vi "Animate two structures.vi"(4 "Atom Size":dbl=0.75, 6 "Scale":dbl(slide)=0.07482993197278912 scale=0.0..0.5, 8 "# Frames":i32(slide)=5 scale=0.0..100.0, 9 "Second Structure":T1, 10 "First Structure":T1, 11 "3D Plot Reference":refnum<vi>) -> ()   [LabVIEW 2010]
uses:
  <vilib>/Analysis/_algsub.llb/Real Vector Norm.vi
  <vilib>/Analysis/NI_AALPro.lvlib
  <vilib>/picture/3D Picture Control/NI_3D Picture Control.lvlib
panel:
  in  "Atomic Structure":refnum<vi>(3d-picture)
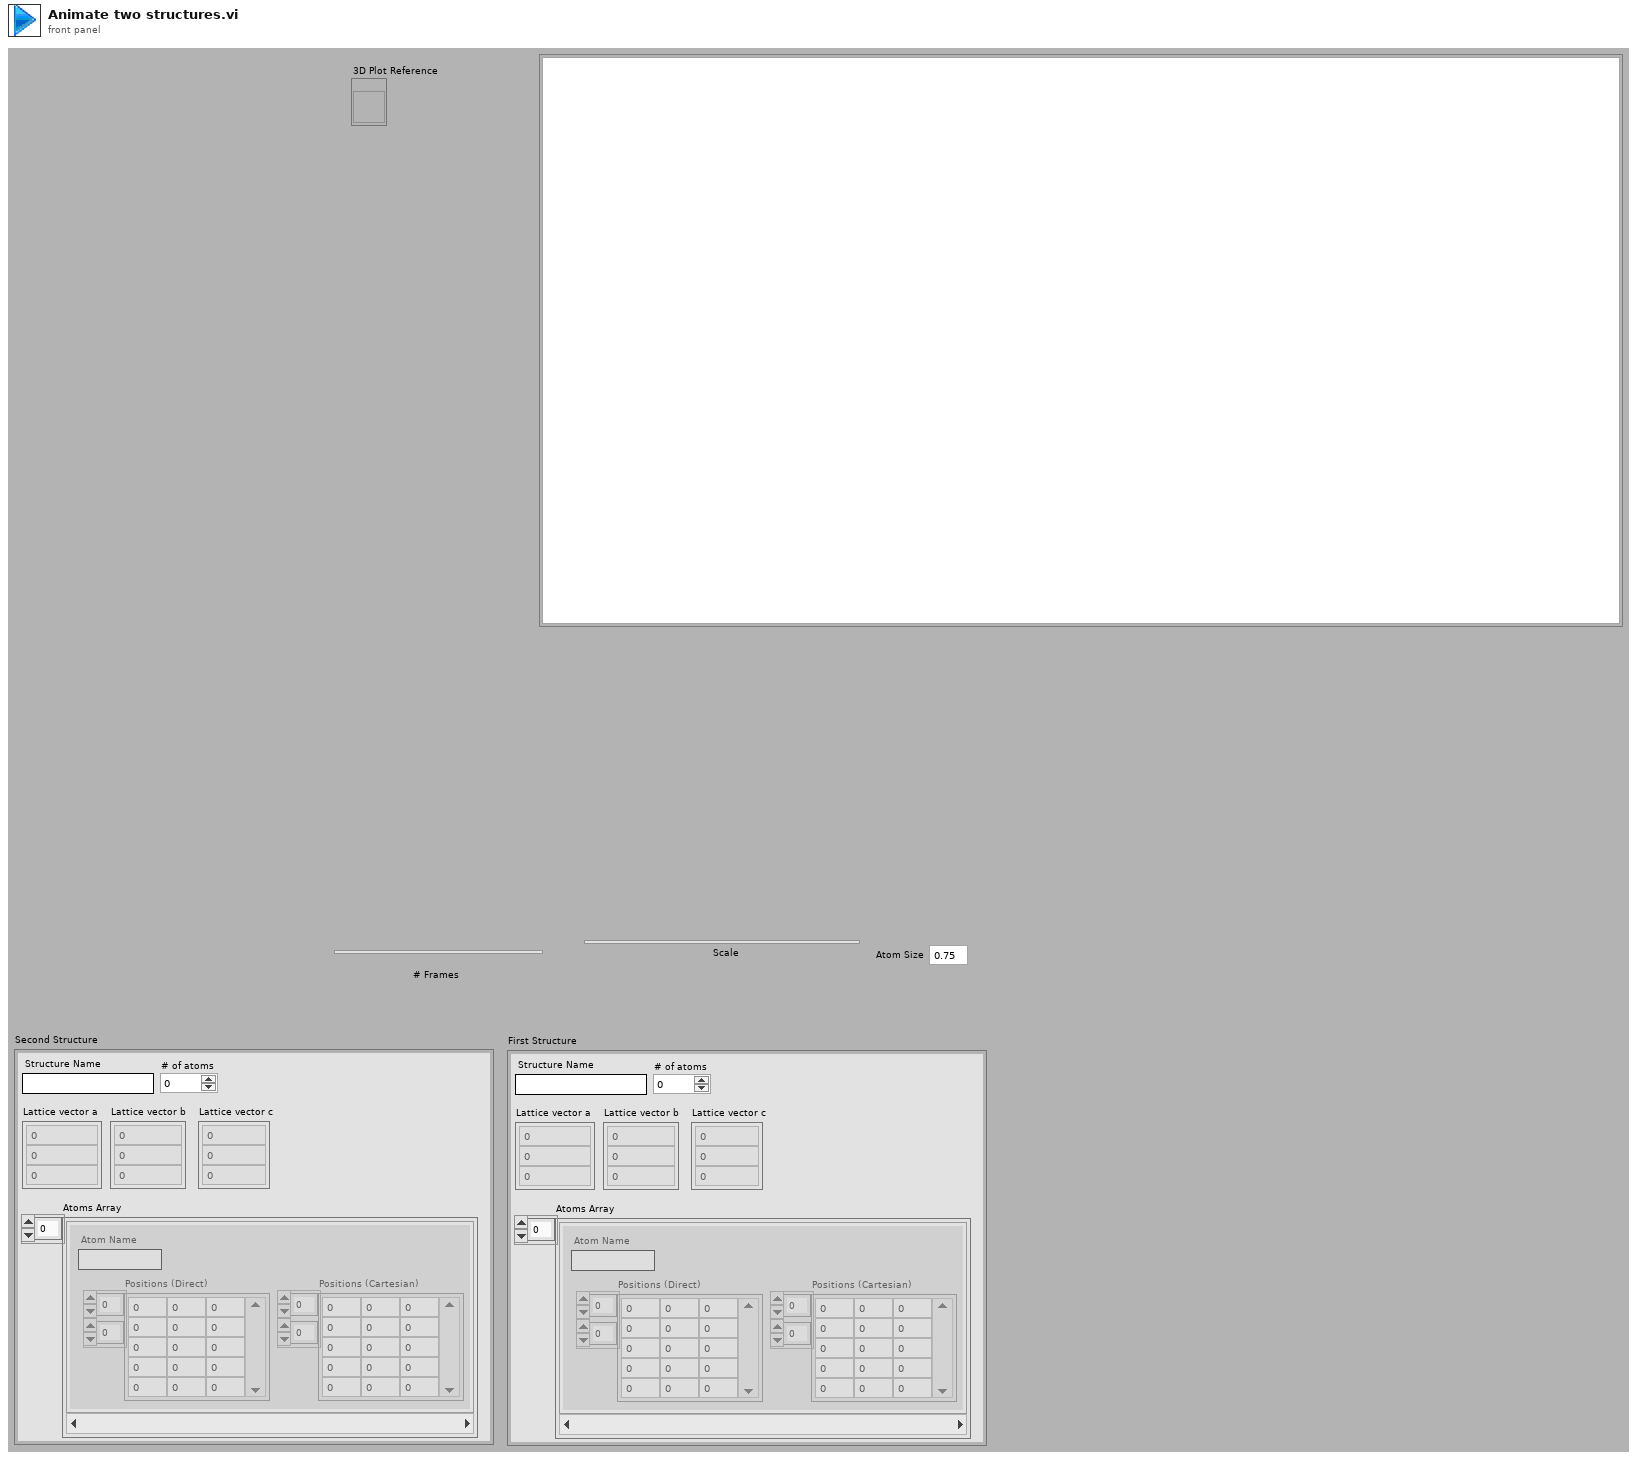
[diagram p1: front panel]
types:
  T1 = cluster{"Structure Name":string, "Lattice vector a":dbl[], "Lattice vector b":dbl[], "Lattice vector c":dbl[], "Atoms Array":cluster{"Atom Name":string, "Positions (Direct)":dbl[][], "Positions (Cartesian)":dbl[][]}[], "# of atoms":i32}
  T2 = cluster{"Red":sgl, "Green":sgl, "Blue":sgl, "Alpha":sgl}[]
  T3 = cluster{"Atom Name":string, "Positions (Direct)":dbl[][], "Positions (Cartesian)":dbl[][]}[]
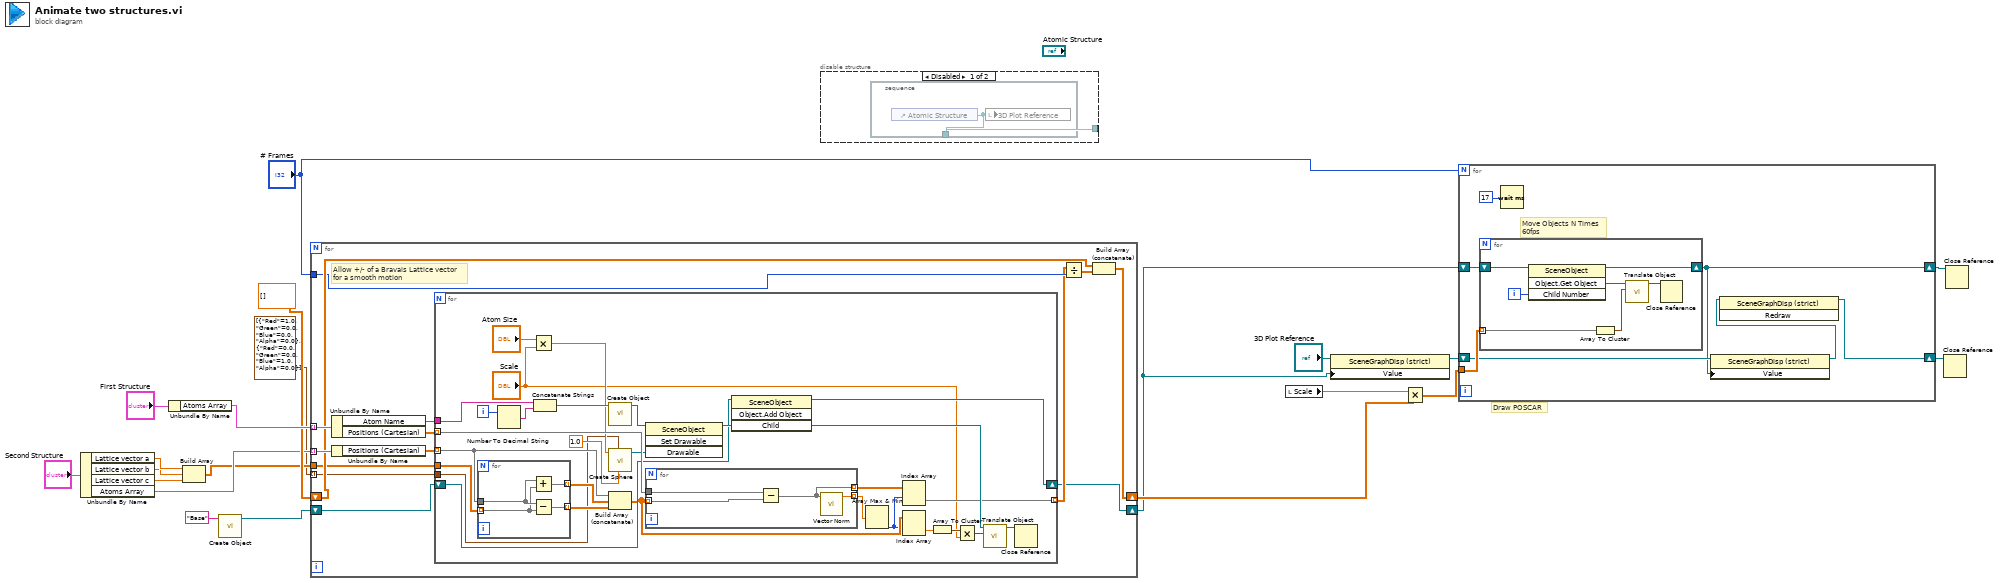
[diagram p0: block diagram]
diagram:
  # "Draw POSCAR"
  n1 = Unbundle By Name("Second Structure") -> ("Lattice vector a"=w15:dbl[], "Lattice vector b"=w14:dbl[], "Lattice vector c"=w13:dbl[], "Atoms Array"=w18:T3)
  n2 = Unbundle By Name("First Structure") -> ("Atoms Array"=w21:T3)
  n3 = Build Array(w15, w14, w13) -> (w12:dbl[][])
  n4 = call <vilib>:"Create Object.vi"("Name"="Base") -> ("Scene:New Object"=w11:refnum<vi>)  [unwired: 1 in, 9 out]
  n5 = for {
    tunnel: w21 -> [w35] mode=indexing
    tunnel: w18 -> [w34] mode=indexing
    shift-right: [w23] -> w9
    shift-left: dbl[][] [] -> [w33]
    tunnel: "# Frames" -> [w32]
    tunnel: w12 -> [w28]
    shift-right: [w22] -> w8
    shift-left: w11 -> [w26]
    tunnel: T2 [{"Red"=1.0, "Green"=0.0, "Blue"=0.0, "Alpha"=0.0}, {"Red"=0.0, "Green"=0.0, "Blue"=1.0, "Alpha"=0.0}] -> [w25] mode=indexing
    # "Allow +/- of a Bravais Lattice vector\nfor a smooth motion"
    n6 = Unbundle By Name(w35) -> ("Atom Name"=w27:string, "Positions (Cartesian)"=w30:dbl[][])
    n7 = Unbundle By Name(w34) -> ("Positions (Cartesian)"=w29:dbl[][])
    n8 = for {
      tunnel: w30 -> [w60] mode=indexing
      tunnel: w29 -> [w63] mode=indexing
      tunnel: w28 -> [w64]
      tunnel: w27 -> [w46]
      shift-right: [w45] -> w22
      shift-left: w26 -> [w44]
      tunnel: w25 -> [w43]
      tunnel: [w42] -> w24 mode=indexing
      i -> [w47]
      n9 = for {
        tunnel: w64 -> [w71] mode=indexing
        tunnel: w63 -> [w72]
        tunnel: [w70] -> w62 mode=indexing
        tunnel: [w69] -> w61 mode=indexing
        n10 = Add(x=w72, y=w71) -> (x+y=w70:dbl[])
        n11 = Subtract(x=w72, y=w71) -> (x-y=w69:dbl[])
      }
      n12 = Number To Decimal String(number=w47) -> (decimal integer string=w56:string)  [unwired: 1 in]
      n13 = Multiply(x="Atom Size", y="Scale") -> (x*y=w49:dbl)
      n14 = Concatenate Strings(w46, w56) -> (w55:string)
      n15 = call <vilib>:"Create Object.vi"("Name"=w55) -> ("Scene:New Object"=w54:refnum<vi>)  [unwired: 1 in, 9 out]
      n16 = call <vilib>:"Create Sphere.vi"("Detail"=sgl 1.0, "Color"=w43, "Radius"=w49) -> ("New Sphere Refnum"=w53:refnum<vi>)  [unwired: 7 in, 1 out]
      n17 = Build Array (concatenate)(w63, w62, w61) -> (w41:dbl[][])
      n18 = invoke class="SceneObject" method="Set Drawable"(reference=w54, "Drawable"=w53) -> (reference out=w52:refnum<vi>)  [unwired: 2 in, 3 out]
      n19 = for {
        tunnel: w41 -> [w68] mode=indexing
        tunnel: w60 -> [w67]
        tunnel: [w66] -> w59 mode=indexing
        tunnel: [w65] -> w58 mode=indexing
        n20 = Subtract(x=w67, y=w68) -> (x-y=w65:dbl[])
        n21 = call-poly <vilib>:"Vector Norm.vi"("Input Vector"=w65) -> ("norm"=w66:dbl)  [unwired: 9 in, 1 out]
      }
      n22 = invoke class="SceneObject" method="Object.Add Object"(reference=w44, "Child"=w52) -> (reference out=w45:refnum<vi>, "Child"=w51:refnum<vi>)  [unwired: 2 in, 2 out]
      n23 = Array Max & Min(array=w59) -> (min index (indices)=w40:i32)  [unwired: 3 out]
      n24 = Index Array(array=w58, index (row)=w40) -> (element=w42:dbl[])  [unwired: 1 in]
      n25 = Index Array(array=w41, index (row)=w40) -> (element=w39:dbl[])  [unwired: 1 in]
      n26 = Array To Cluster(array=w39) -> (cluster=w50:cluster{"[0]":dbl, "[1]":dbl, "[2]":dbl})
      n27 = Multiply(x=w50, y="Scale") -> (x*y=w48:cluster{"[0]":dbl, "[1]":dbl, "[2]":dbl})
      n28 = call <vilib>:"Translate Object.vi"("Translation"=w48, "Scene.Object In"=w51) -> ("Scene.Object Out"=w38:refnum<vi>)  [unwired: 1 in, 8 out]
      n29 = Close Reference(reference=w38) -> ()  [unwired: 1 in, 1 out]
    }
    n30 = Divide(x=w24, y=w32) -> (x/y=w31:dbl[][])
    n31 = Build Array (concatenate)(w33, w31) -> (w23:dbl[][])
  }
  n32 = disable-structure shown="Disabled" {
    disable-tunnel: [w73 _] -> _
    frame Disabled {
      n33 = stacked-sequence {
        tunnel: [w74] -> w73
        frame #0 {
          n34 = control-ref of="Atomic Structure"() -> (w74:refnum<vi>)
          n35 = local write "3D Plot Reference"(w74) -> ()
        }
      }
    }
    frame Enabled {
    }
  }
  n36 = local read "Scale"() -> (w2:dbl)
  n37 = property class="SceneGraphDisp (strict)"(reference="3D Plot Reference", "Value"=w8) -> (reference out=w5:refnum<vi>)  [unwired: 1 in, 1 out]
  n38 = Multiply(x=w2, y=w9) -> (x*y=w16:dbl[][])
  n39 = for {
    N: "# Frames" -> [_]
    tunnel: w16 -> [w81]
    shift-right: [w77] -> w3
    shift-left: w8 -> [w80]
    shift-right: [w75] -> w4
    shift-left: w5 -> [w78]
    # "Move Objects N Times\n60fps"
    n40 = for {
      tunnel: w81 -> [w87] mode=indexing
      shift-right: [w86] -> w77
      shift-left: w80 -> [w85]
      i -> [w88]
      n41 = invoke class="SceneObject" method="Object.Get Object"(reference=w85, "Child Number"=w88) -> (reference out=w86:refnum<vi>, "Get Child"=w84:refnum<vi>)  [unwired: 2 in, 2 out]
      n42 = Array To Cluster(array=w87) -> (cluster=w83:cluster{"[0]":dbl, "[1]":dbl, "[2]":dbl})
      n43 = call <vilib>:"Translate Object.vi"("Translation"=w83, "Scene.Object In"=w84) -> ("Scene.Object Out"=w82:refnum<vi>)  [unwired: 1 in, 8 out]
      n44 = Close Reference(reference=w82) -> ()  [unwired: 1 in, 1 out]
    }
    n45 = Wait (ms)(milliseconds to wait=u32 17) -> ()  [unwired: 1 out]
    n46 = property class="SceneGraphDisp (strict)"(reference=w78, "Value"=w77) -> (reference out=w76:refnum<vi>)  [unwired: 1 in, 1 out]
    n47 = invoke on="Invoke Node" class="SceneGraphDisp (strict)" method="Redraw"(reference=w76) -> (reference out=w75:refnum<vi>)  [unwired: 2 in, 2 out]
  }
  n48 = Close Reference(reference=w4) -> ()  [unwired: 1 in, 1 out]
  n49 = Close Reference(reference=w3) -> ()  [unwired: 1 in, 1 out]
